vi "steer test.vi"() -> ()   [LabVIEW 2013]
uses:
  <vilib>/NXT/Block Support/NXT_InputPort.ctl
  <vilib>/NXT/Subs/MotorOutput.ctl
panel:
  out "Steering (100)":i32=-10
  in  "threshold steer":dbl=0.2
  out "norm dist":dbl
  out "right dist":i16
  out "left dist":i16
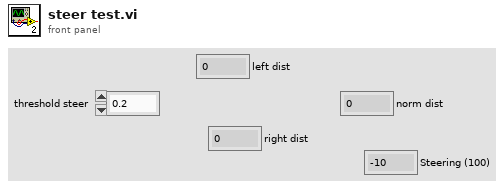
[diagram p1: front panel]
types:
  T1 = typedef "NXT_InputPort.ctl" = u32
  T2 = typedef "LVHSConnector.ctl" = refnum<class "BrickReference.lvclass">
  T3 = typedef "MotorOutput.ctl" = u8
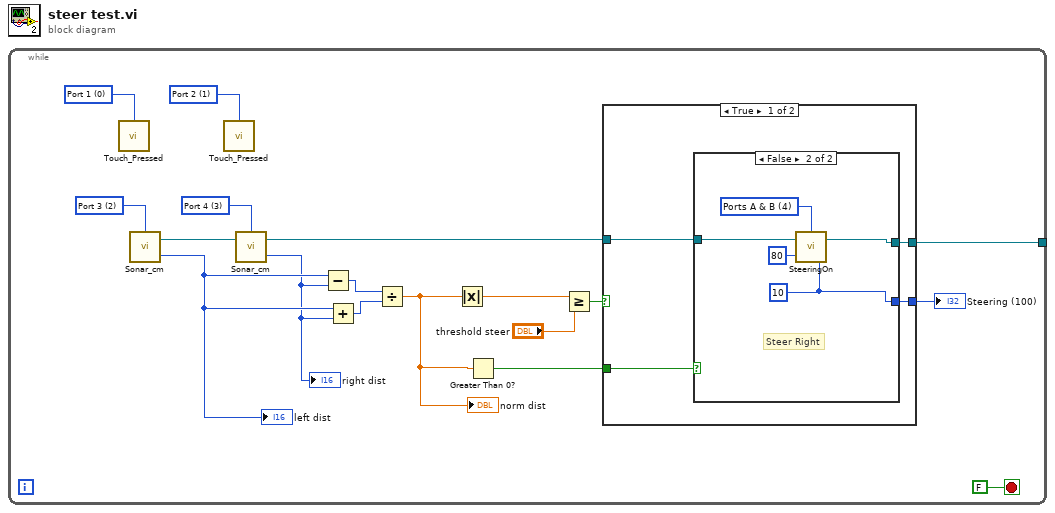
[diagram p0: block diagram]
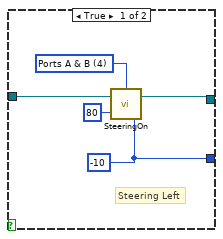
[diagram p2: hidden frame]
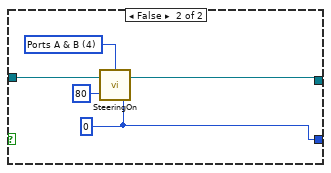
[diagram p3: hidden frame]
diagram:
  n1 = while {
    tunnel: [w5] -> _
    stop <- FALSE stop-if-true
    w1 = T1 1 items=["Port 1", "Port 2", "Port 3", "Port 4"] ("Port (Port 1)")
    w2 = T1 0 items=["Port 1", "Port 2", "Port 3", "Port 4"] ("Port (Port 1)")
    w17 = T1 3 items=["Port 1", "Port 2", "Port 3", "Port 4"] ("Port (Port 4)")
    w18 = T1 2 items=["Port 1", "Port 2", "Port 3", "Port 4"] ("Port (Port 4)")
    n2 = call <vilib>:"Touch_Pressed.vi"("Port (Port 1)"=w2) -> ()  [unwired: 2 in, 2 out]
    n3 = call <vilib>:"Sonar_cm.vi"("Port (Port 4)"=w18) -> ("Distance (cm)"=w15:i16, "NXT/EV3"=w16:T2)  [unwired: 2 in]
    "left dist" <- w15
    n4 = call <vilib>:"Touch_Pressed.vi"("Port (Port 1)"=w1) -> ()  [unwired: 2 in, 2 out]
    n5 = call <vilib>:"Sonar_cm.vi"("NXT/EV3"=w16, "Port (Port 4)"=w17) -> ("Distance (cm)"=w14:i16, "NXT/EV3"=w8:T2)  [unwired: 1 in]
    "right dist" <- w14
    n6 = Subtract(x=w15, y=w14) -> (x-y=w13:i16)
    n7 = Add(x=w15, y=w14) -> (x+y=w12:i16)
    n8 = Divide(x=w13, y=w12) -> (x/y=w7:dbl)
    "norm dist" <- w7
    n9 = Absolute Value(x=w7) -> (abs(x)=w11:dbl)
    n10 = Greater Than 0?(x=w7) -> (x > 0?=w6:bool)
    n11 = Greater Or Equal?(x=w11, y="threshold steer") -> (x >= y?=w9:bool)
    n12 = case shown="True" w9 {
      tunnel: w8 -> [w22 w37]
      tunnel: w6 -> [w21 _]
      tunnel: [w20 w34] -> w5
      tunnel: [w19 w33] -> w3
      frame True {
        n13 = case shown="False" w21 {
          tunnel: w22 -> [w27 w32]
          tunnel: [w24 w29] -> w20
          tunnel: [w23 w28] -> w19
          frame True {
            w23 = -10 ("Steering (100)")
            w26 = T3 4 items=["Port A"=0, "Port B"=1, "Port C"=2, "Ports A & B"=4, "Ports A & C"=5, "Ports B & C"=6, "All Ports"=3] ("Output Ports (A & B)")
            # "Steering Left"
            n14 = call <vilib>:"SteeringOn.vi"("Power (75)"=80, "Steering (100)"=w23, "NXT/EV3"=w27, "Output Ports (A & B)"=w26) -> ("NXT/EV3"=w24:T2)
          }
          frame False {
            w28 = 10 ("Steering (100)")
            w31 = T3 4 items=["Port A"=0, "Port B"=1, "Port C"=2, "Ports A & B"=4, "Ports A & C"=5, "Ports B & C"=6, "All Ports"=3] ("Output Ports (A & B)")
            # "Steer Right"
            n15 = call <vilib>:"SteeringOn.vi"("Power (75)"=80, "Steering (100)"=w28, "NXT/EV3"=w32, "Output Ports (A & B)"=w31) -> ("NXT/EV3"=w29:T2)
          }
        }
      }
      frame False {
        w33 = 0 ("Steering (100)")
        w36 = T3 4 items=["Port A"=0, "Port B"=1, "Port C"=2, "Ports A & B"=4, "Ports A & C"=5, "Ports B & C"=6, "All Ports"=3] ("Output Ports (A & B)")
        n16 = call <vilib>:"SteeringOn.vi"("Power (75)"=80, "Steering (100)"=w33, "NXT/EV3"=w37, "Output Ports (A & B)"=w36) -> ("NXT/EV3"=w34:T2)
      }
    }
    "Steering (100)" <- w3
  }
